vi "SupplyDatenBundle (SubVI).vi"(9 "dt":dbl, 10 "SupplyStrom":dbl[](array[numeric]), 11 "SupplySpannung":dbl[](array[numeric])) -> (1 "Supply Current":waveform(dbl), 2 "Supply Voltage":waveform(dbl), 3 "Supply Output":T1 {"Current mean" format="%0.4f"; "Voltage mean" format="%0.2f"})   [LabVIEW 2018]
uses:
  Type/SupplyOutput.ctl
  <vilib>/Analysis/baseanly.llb/Mean (DBL).vi
  <vilib>/Analysis/NI_AALBase.lvlib
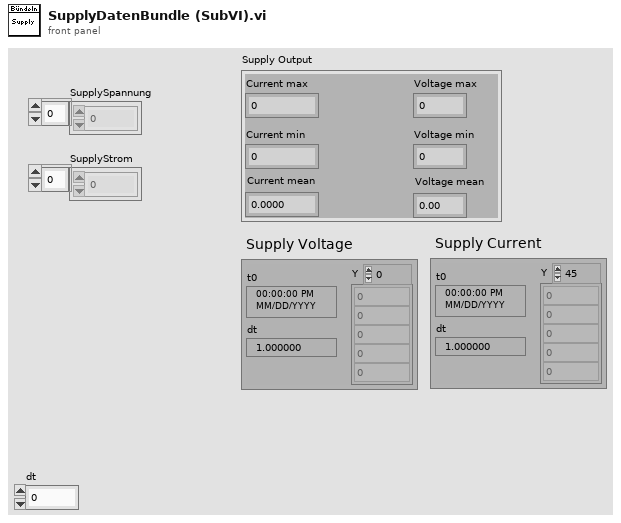
[diagram p1: front panel]
types:
  T1 = typedef "SupplyOutput.ctl" = cluster{"Current max":dbl, "Current min":dbl, "Voltage max":dbl, "Voltage min":dbl, "Voltage mean":dbl, "Current mean":dbl}
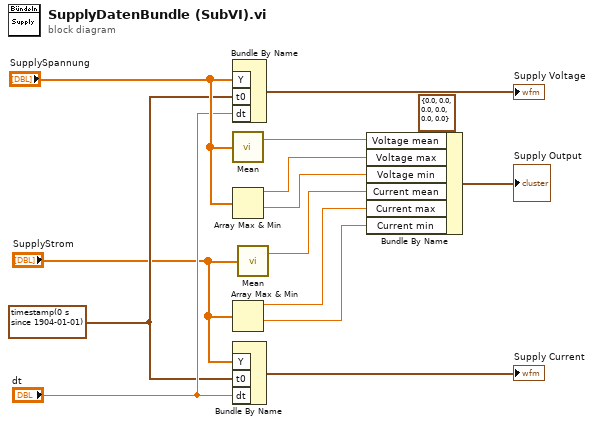
[diagram p0: block diagram]
diagram:
  w3 = timestamp(0 s since 1904-01-01) ("Zeitstempel")
  n1 = Bundle By Name("Y"="SupplySpannung", "t0"=w3, "dt"="dt") -> (→"Supply Voltage":waveform(dbl))  [unwired: 1 in]
  n2 = call-poly <vilib>:"Mean.vi"("X"="SupplySpannung") -> ("mean"=w9:dbl)  [unwired: 1 out]
  n3 = Array Max & Min(array="SupplySpannung") -> (max value=w10:dbl, min value=w11:dbl)  [unwired: 2 out]
  n4 = Array Max & Min(array="SupplyStrom") -> (max value=w13:dbl, min value=w14:dbl)  [unwired: 2 out]
  n5 = Bundle By Name("Y"="SupplyStrom", "t0"=w3, "dt"="dt") -> (→"Supply Current":waveform(dbl))  [unwired: 1 in]
  n6 = call-poly <vilib>:"Mean.vi"("X"="SupplyStrom") -> ("mean"=w12:dbl)  [unwired: 1 out]
  n7 = Bundle By Name(cluster=T1 {"Current max"=0.0, "Current min"=0.0, "Voltage max"=0.0, "Voltage min"=0.0, "Voltage mean"=0.0, "Current mean"=0.0} ("Supply Output 2"), "Voltage mean"=w9, "Voltage max"=w10, "Voltage min"=w11, "Current mean"=w12, "Current max"=w13, "Current min"=w14) -> (→"Supply Output":T1)
